vi "Pump2 data.vi"(4 "P3":dbl format="%.2f", 5 "P2":dbl format="%.2f", 7 "Volume PV":dbl format="%.2f", 8 "error in":errorcluster, 9 "Flow PV":dbl format="%#.6f", 10 "Pressure PV":dbl format="%.3f") -> (0 "error out":errorcluster)   [LabVIEW 2023, in "Drive.lvlib"]
doc: "_____\nCreated using DQMH Event Scripter 7.0.1.1316."
uses:
  Drive.lvlib
  Pump2 data Argument--cluster.ctl
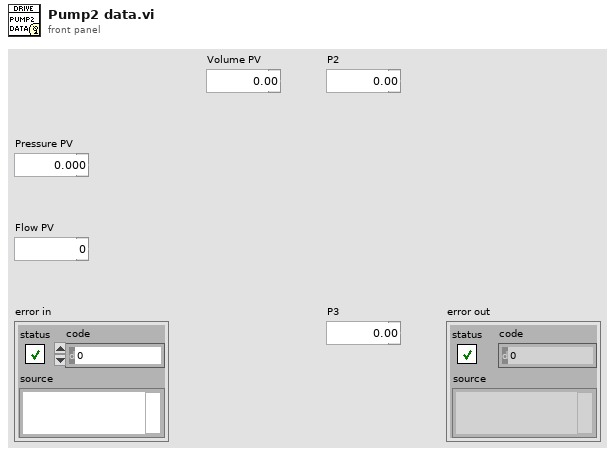
[diagram p1: front panel]
types:
  T1 = typedef "Drive.lvlib/Pump2 data Argument--cluster.ctl" = cluster{"Pressure PV":dbl, "Flow PV":dbl, "Volume PV":dbl, "P2":dbl, "P3":dbl}
  T2 = typedef "Drive.lvlib/Broadcast Events--cluster.ctl" = cluster{"Module Did Init":refnum<user-event>, "Status Updated":refnum<user-event>, "Error Reported":refnum<user-event>, "Module Did Stop":refnum<user-event>, "Update Module Execution Status":refnum<user-event>, "Pump_Data":refnum<user-event>, "Rotate Data":refnum<user-event>, "Pump2 data":refnum<user-event>}
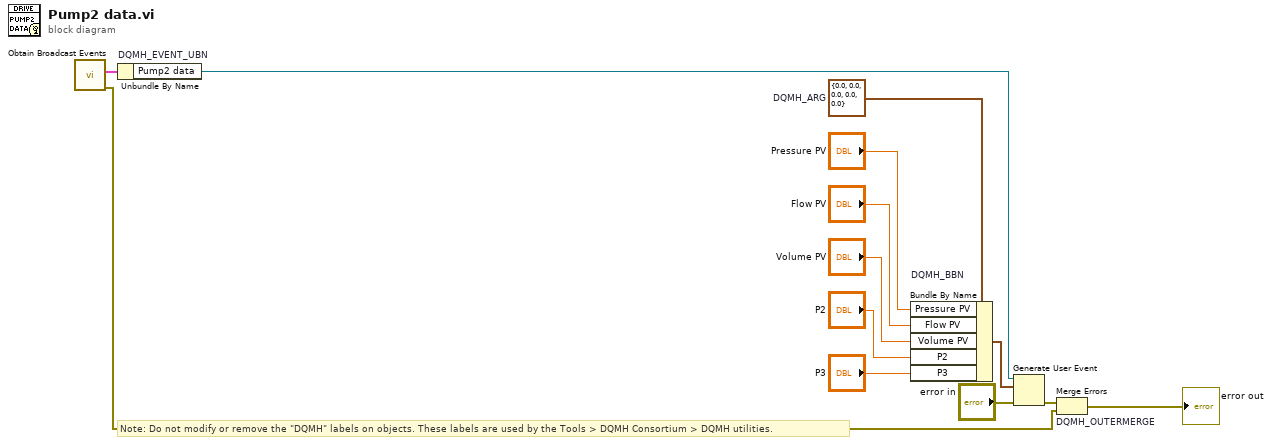
[diagram p0: block diagram]
diagram:
  w8 = T1 {"Pressure PV"=0.0, "Flow PV"=0.0, "Volume PV"=0.0, "P2"=0.0, "P3"=0.0}  # DQMH_ARG
  # "Note: Do not modify or remove the \"DQMH\" labels on objects. These labels are used by the Tools > DQMH Consortium > DQMH utilities."
  n1 = call "Obtain Broadcast Events.vi"() -> ("error out"=w2:errorcluster, "Drive Broadcast Events"=w1:T2)  [unwired: 10 in]
  n2 = Unbundle By Name "DQMH_EVENT_UBN"(w1) -> ("Pump2 data"=w10:refnum<user-event>)
  n3 = Bundle By Name "DQMH_BBN"(cluster=w8, "Pressure PV"="Pressure PV", "Flow PV"="Flow PV", "Volume PV"="Volume PV", "P2"="P2", "P3"="P3") -> (w11:T1)
  n4 = Generate User Event(user event=w10, event data cluster=w11, error in="error in") -> (error out=w9:errorcluster)  [unwired: 1 in, 1 out]
  n5 = Merge Errors "DQMH_OUTERMERGE"(w9, w2) -> (→"error out":errorcluster)
